vi "mean-e-ficator.vi"(6 "first time":bool=TRUE, 7 "size":i32=1, 11 "number":cdb) -> (2 "mean":cdb)   [LabVIEW 2010]
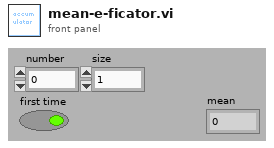
[diagram p1: front panel]
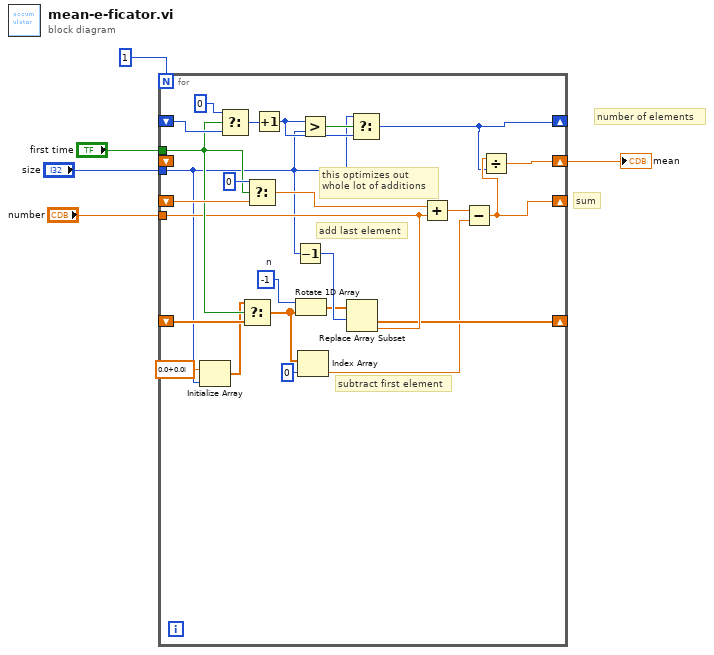
[diagram p0: block diagram]
diagram:
  # "sum"
  # "number of elements"
  n1 = for {
    N: 1 -> [_]
    tunnel: "first time" -> [w22]
    shift-right: [w8] -> _
    shift-left: _ -> [w26]
    shift-right: [w7] -> _
    shift-left: _ -> [w29]
    tunnel: "size" -> [w9]
    tunnel: "number" -> [w19]
    shift-right: [w16] -> _
    shift-left: _ -> [w21]
    shift-right: [w6] -> w1
    shift-left: _ -> [_]
    w20 = -1  # n
    # "add last element"
    # "subtract first element"
    # "this optimizes out \nwhole lot of additions"
    n2 = Initialize Array(cdb 0.0+0.0i, w9) -> (w10:cdb[])
    n3 = Select(t=0, s=w22, f=w29) -> (s? t:f=w24:i32)
    n4 = Select(t=w10, s=w22, f=w21) -> (s? t:f=w13:cdb[])
    n5 = Select(t=0, s=w22, f=w26) -> (s? t:f=w25:cdb)
    n6 = Increment(x=w24) -> (x+1=w23:i32)
    n7 = Decrement(x=w9) -> (x-1=w18:i32)
    n8 = Rotate 1D Array(1:w13, 2:w20) -> (0:w17:cdb[])
    n9 = Index Array(array=w13, index=0) -> (element=w12:cdb)
    n10 = Greater?(x=w23, y=w9) -> (0:w28:bool)
    n11 = Replace Array Subset(array=w17, new element=w19, index=w18) -> (w16:cdb[])
    n12 = Select(t=w9, s=w28, f=w23) -> (s? t:f=w7:i32)
    n13 = Add(x=w25, y=w19) -> (x+y=w15:cdb)
    n14 = Subtract(x=w15, y=w12) -> (x-y=w8:cdb)
    n15 = Divide(x=w8, y=w7) -> (x/y=w6:cdb)
  }
  "mean" <- w1
